vi "Draw(1).vi"(8 "error in (no error)":errorcluster, 10 "Picture in":picture, 11 "Triangle in":refnum<class "Triangle.lvclass">) -> (0 "error out":errorcluster, 2 "Picture out":picture, 3 "Triangle out":refnum<class "Triangle.lvclass">)   [LabVIEW 2015, in "Triangle.lvclass"]
uses:
  Triangle.lvclass
  Interfaces/Shape/Shape.lvclass/Shape.ctl
  Interfaces/Shape/Shape.lvclass
panel:
  # "NOTICE -- YOU MUST LEAVE THIS NOTICE IN PLACE.\n\nCopyright (c) 2017, LIANG LIU Shawn.Liu.cn@gmail.com\nAll rights reserved.\n\nRedistribution and use in source and binary forms, with or without modification, are permitted provided that the following conditions are met:\n-Redistributions of source code must retain the above copyright notice, this list of conditions and the following disclaimer.\n-Redistributions in binary form must reproduce the above copyright notice, this list of conditions and the following disclaimer in the documentation and/or other materials provided with the distribution.\n-Neither the name of the eLp nor the names of its contributors may be used to endorse or promote products derived from this software without specific prior written permission.\n\nTHIS SOFTWARE IS PROVIDED BY THE COPYRIGHT HOLDERS AND CONTRIBUTORS \"AS IS\" AND ANY EXPRESS OR IMPLIED WARRANTIES, INCLUDING, BUT NOT LIMITED TO, THE IMPLIED WARRANTIES OF MERCHANTABILITY AND FITNESS FOR A PARTICULAR PURPOSE ARE DISCLAIMED. IN NO EVENT SHALL THE COPYRIGHT HOLDER OR CONTRIBUTORS BE LIABLE FOR ANY DIRECT, INDIRECT, INCIDENTAL, SPECIAL, EXEMPLARY, OR CONSEQUENTIAL DAMAGES (INCLUDING, BUT NOT LIMITED TO, PROCUREMENT OF SUBSTITUTE GOODS OR SERVICES; LOSS OF USE, DATA, OR PROFITS; OR BUSINESS INTERRUPTION) HOWEVER CAUSED AND ON ANY THEORY OF LIABILITY, WHETHER IN CONTRACT, STRICT LIABILITY, OR TORT (INCLUDING NEGLIGENCE OR OTHERWISE) ARISING IN ANY WAY OUT OF THE USE OF THIS SOFTWARE, EVEN IF ADVISED OF THE POSSIBILITY OF SUCH DAMAGE."
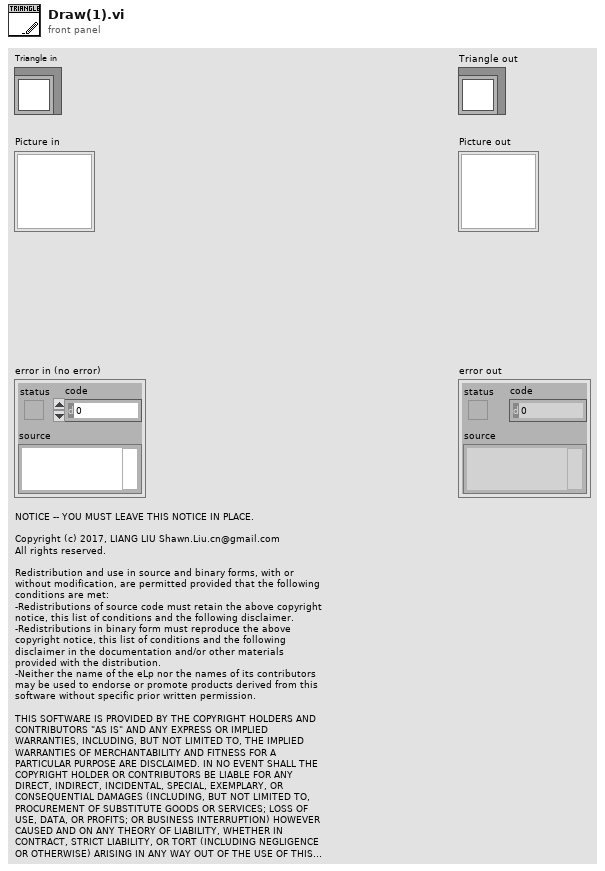
[diagram p1: front panel]
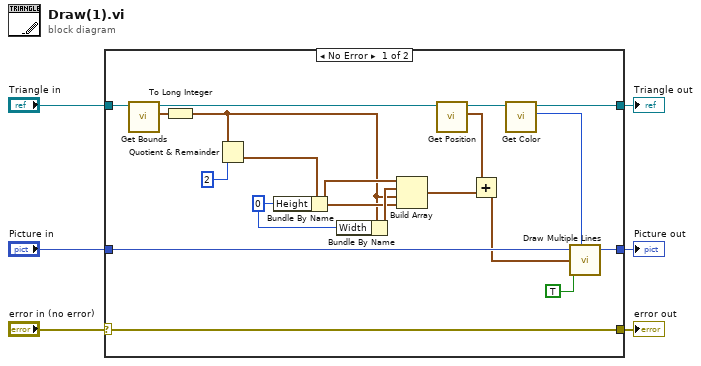
[diagram p0: block diagram]
diagram:
  n1 = case shown="No Error" "error in (no error)" {
    selector: "error in (no error)" -> [w25 w28]
    tunnel: "Triangle in" -> [w24 w27]
    tunnel: [w12 w26] -> w4
    tunnel: "Picture in" -> [w11 w26]
    tunnel: [w9 w27] -> w2
    tunnel: [w25 w28] -> w1
    frame No Error {
      w19 = 0 ("Height")
      n2 = call "Get Bounds.vi"("Shape in"=w24) -> ("Bounds"=w14:cluster{"Width":u32, "Height":u32}, "Shape out"=w23:refnum<class "Triangle.lvclass">)  [unwired: 9 in]
      n3 = To Long Integer(number=w14) -> (32bit integer=w13:cluster{"Width":i32, "Height":i32})
      n4 = Quotient & Remainder(x=w13, y=2) -> (floor(x/y)=w21:cluster{"Width":i32, "Height":i32})  [unwired: 1 out]
      n5 = Bundle By Name(cluster=w21, "Height"=w19) -> (w17:cluster{"Width":i32, "Height":i32})
      n6 = Bundle By Name(cluster=w13, "Width"=w19) -> (w18:cluster{"Width":i32, "Height":i32})
      n7 = Build Array(w17, w18, w13, w17) -> (w16:cluster{"Width":i32, "Height":i32}[])
      n8 = call "Get Position.vi"("Shape in"=w23) -> ("Position"=w15:cluster{"Left":i32, "Top":i32}, "Shape out"=w22:refnum<class "Triangle.lvclass">)  [unwired: 9 in]
      n9 = Add(x=w15, y=w16) -> (x+y=w10:cluster{i32, i32}[])
      n10 = call "Get Color.vi"("Shape in"=w22) -> ("Color"=w8:u32, "Shape out"=w9:refnum<class "Triangle.lvclass">)  [unwired: 9 in]
      n11 = call <vilib>:"Draw Multiple Lines.vi"("picture"=w11, "line endpoints"=w10, "fill?(F)"=TRUE, "color(black)"=w8) -> ("new picture"=w12:picture)  [unwired: 5 in]
    }
    frame Error {
    }
  }
  "error out" <- w1
  "Triangle out" <- w2
  "Picture out" <- w4
